vi "SUB_ASKLEDS_AllOff.vi"() -> (1 "yes/no":enum32{"No Selection", "Yes", "No", "None"}(ring))   [LabVIEW 2011]
doc: "This is an example of how to use the radio buttons control with the Value Changed event."
panel:
  in  "Answer Question":enum32{"No Selection", "Yes", "No", "None"}(radio)=enum."Yes"
  # "4ÁûLED³£·À(¤£«G)?"
  # "NG"
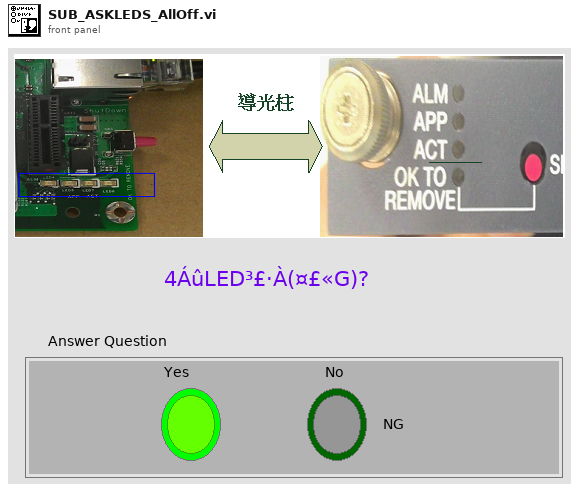
[diagram p1: front panel]
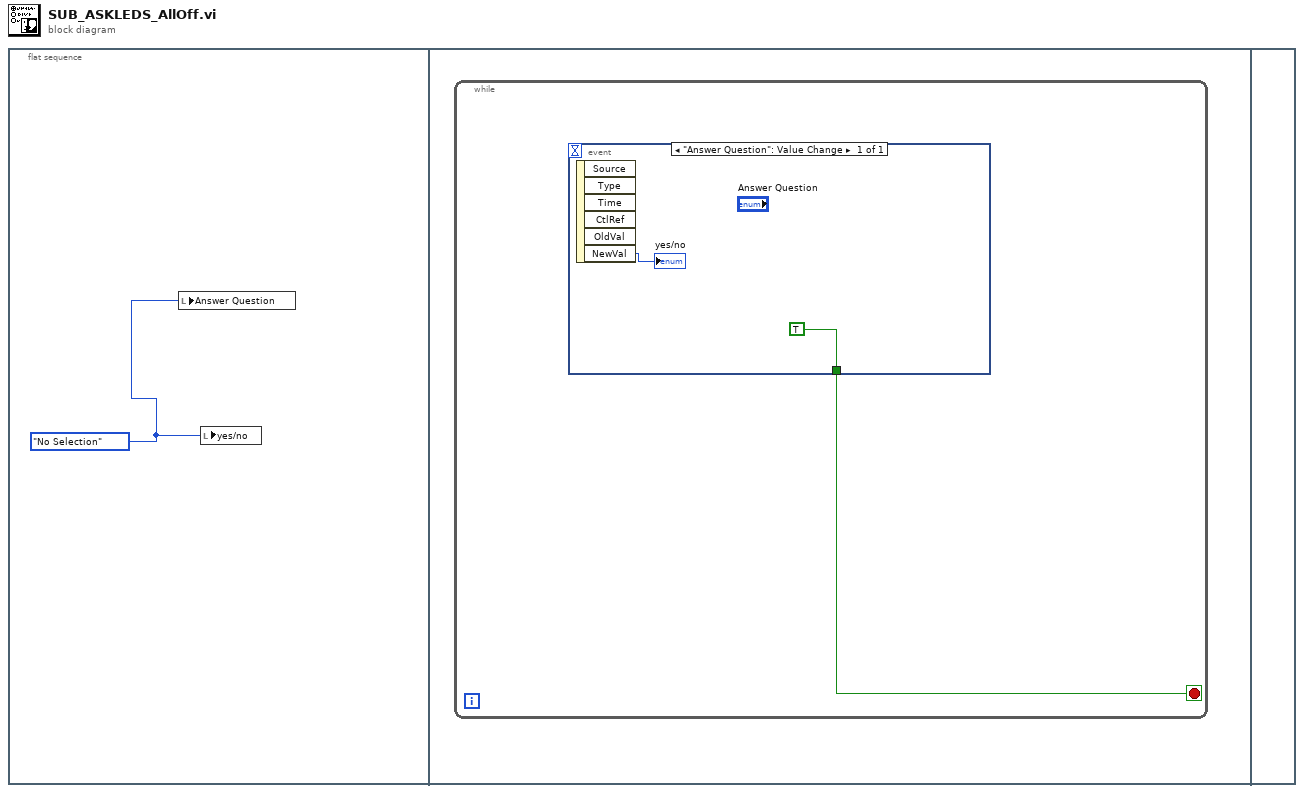
[diagram p0: block diagram]
diagram:
  n1 = flat-sequence {
    frame #0 {
      w1 = enum32{"No Selection", "Yes", "No", "None"}."No Selection" ("yes/no")
      n2 = local write "Answer Question"(w1) -> ()
      n3 = local write "yes/no"(w1) -> ()
    }
    frame #1 {
      n4 = while {
        stop <- w2 stop-if-true
        n5 = event shown="[0] \"Answer Question\": Value Change" {
          selector: _ -> [_]
          dyn-events: _ -> [_]
          timeout: _ -> [_]
          tunnel: [TRUE] -> w2
          event "Answer Question": Value Change {
            n6 = event-data() -> ("NewVal"=→"yes/no":enum32{"No Selection", "Yes", "No", "None"})  [unwired: 1 in, 5 out]
          }
        }
      }
    }
    frame #2 {
    }
  }
